vi "FL_Gen_Bins_for_RunLengths.vi"(2 "Min run, m":dbl=0.2 format="%#_13g", 3 "N bins":u16=10, 4 "Max run, m":dbl=2.0 format="%#_13g") -> (1 "Bins array":dbl[](array[numeric])=[0.0, 8.0, 44.5, 81.0, 117.5, 154.0, 190.5, 227.0, 263.5, 300.0, inf])   [LabVIEW 2018, in "Tracker.lvlib"]
uses:
  Tracker.lvlib
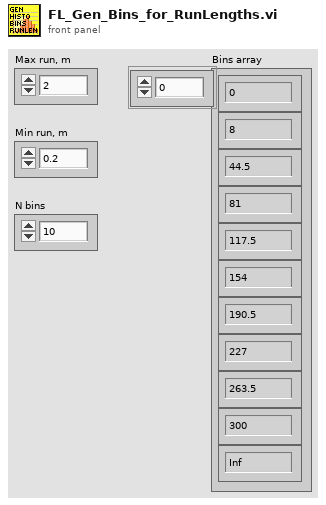
[diagram p1: front panel]
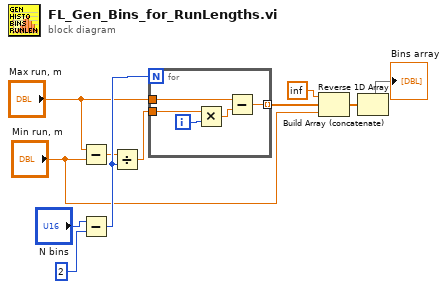
[diagram p0: block diagram]
diagram:
  n1 = Subtract(x="Max run, m", y="Min run, m") -> (x-y=w6:dbl)
  n2 = Subtract(x="N bins", y=u16 2) -> (x-y=w8:u16)
  n3 = Divide(x=w6, y=w8) -> (x/y=w7:dbl)
  n4 = for {
    N: w8 -> [_]
    tunnel: "Max run, m" -> [w16]
    tunnel: w7 -> [w15]
    tunnel: [w14] -> w9 mode=indexing
    i -> [w12]
    n5 = Multiply(x=w15, y=w12) -> (x*y=w13:dbl)
    n6 = Subtract(x=w16, y=w13) -> (x-y=w14:dbl)
  }
  n7 = Build Array (concatenate)(inf, w9, "Min run, m") -> (w10:dbl[])
  n8 = Reverse 1D Array(array=w10) -> (reversed array=→"Bins array":dbl[])
